vi "AWG Close.vi"(8 "error in (no error)":errorcluster, 11 "awg session in":T1) -> (0 "error out":errorcluster, 3 "awg session out":T1)   [LabVIEW 2013, in "AWG.lvlib"]
doc: "AWG wrapper: close function generator. Returns AWG to local control."
uses:
  AWG.lvlib
  AWG Session.ctl
  AWG Type.ctl
  <vilib>/Instr/_visa.llb/VISA GPIB Control REN Mode.ctl
  Agilent 33XXX Series/Agilent 33XXX Series.lvlib
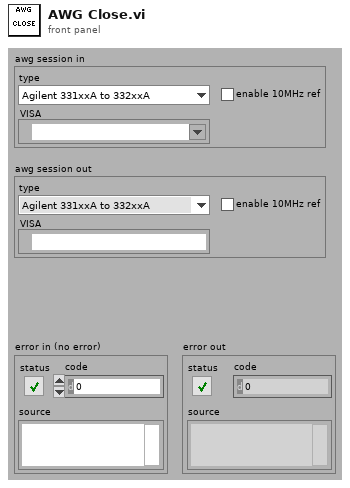
[diagram p1: front panel]
types:
  T1 = typedef "AWG.lvlib/AWG Session.ctl" = cluster{"type":T2, "VISA":refnum<visa-resource-name>, "enable 10MHz ref":bool}
  T2 = typedef "AWG.lvlib/AWG Type.ctl" = enum16{"Agilent 331xxA to 332xxA", "Agilent 335xxA to 336xxA", "dummy"}
  T3 = typedef "VISA GPIB Control REN Mode.ctl" = u16
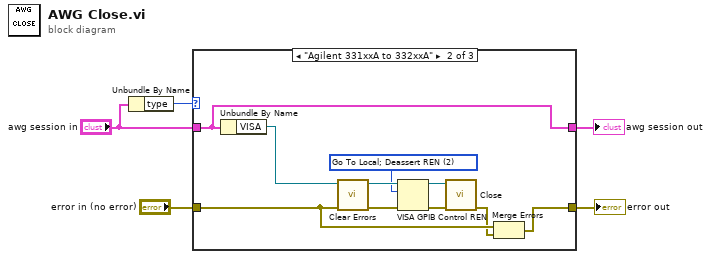
[diagram p0: block diagram]
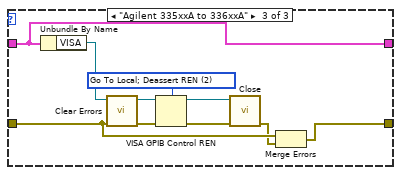
[diagram p3: hidden frame]
diagram:
  n1 = Unbundle By Name("awg session in") -> ("type"=w5:T2)
  n2 = case shown="\"Agilent 331xxA to 332xxA\"" w5 {
    tunnel: "error in (no error)" -> [w7 w11 w19]
    tunnel: [w7 w8 w17] -> w3
    tunnel: "awg session in" -> [w6 w16 w25]
    tunnel: [w6 w16 w25] -> w1
    frame Default {
    }
    frame "Agilent 331xxA to 332xxA" {
      w14 = T3 2 items=["Deassert REN", "Assert REN", "Go To Local; Deassert REN ", "Assert REN; Address Device", "Local Lockout (Addressed Devices)", "Local Lockout (This Device)", "Go To Local"] ("Mode")
      n3 = Unbundle By Name(w16) -> ("VISA"=w15:refnum<visa-resource-name>)
      n4 = call <vilib>:"Clear Errors.vi"("error in (no error)"=w11) -> ("error out"=w12:errorcluster)  [unwired: 6 in]
      n5 = VISA GPIB Control REN(8:w12, 10:w14, 11:w15) -> (0:w10:errorcluster, 3:w13:refnum<visa-resource-name>)
      n6 = call "Close.vi"("error in (no error)"=w10, "VISA resource name"=w13) -> ("error out"=w9:errorcluster)  [unwired: 9 in]
      n7 = Merge Errors(w11, w9) -> (w8:errorcluster)
    }
    frame "Agilent 335xxA to 336xxA" {
      w21 = T3 2 items=["Deassert REN", "Assert REN", "Go To Local; Deassert REN ", "Assert REN; Address Device", "Local Lockout (Addressed Devices)", "Local Lockout (This Device)", "Go To Local"] ("Mode")
      n8 = Unbundle By Name(w25) -> ("VISA"=w23:refnum<visa-resource-name>)
      n9 = call <vilib>:"Clear Errors.vi"("error in (no error)"=w19) -> ("error out"=w20:errorcluster)  [unwired: 6 in]
      n10 = VISA GPIB Control REN(8:w20, 10:w21, 11:w23) -> (0:w24:errorcluster, 3:w22:refnum<visa-resource-name>)
      n11 = call "Close.vi"("error in (no error)"=w24, "VISA resource name"=w22) -> ("error out"=w18:errorcluster)  [unwired: 9 in]
      n12 = Merge Errors(w19, w18) -> (w17:errorcluster)
    }
  }
  "error out" <- w3
  "awg session out" <- w1
